vi "Errors.vi"   [LabVIEW 2017, in "Memory Manager.lvlib" / "Protected Pointer.lvclass"]
uses:
  Protected Pointer.lvclass
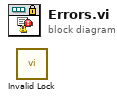
[diagram p0: block diagram]
diagram:
  n1 = call "Invalid Lock.vi"() -> ()  [unwired: 10 in, 2 out]
